vi "Time series ini AVI & header file.vi"(8 "error in (no error)":errorcluster) -> (0 "error out":errorcluster)   [LabVIEW 2017]
uses:
  Typedefs/Channel Selector.ctl
  Global Variables/General Globals.vi
  User Interface/Visualisation/Functional Imaging Viewer/SubVIs/Experiment header interface/Typedefs/Header file type enum.ctl
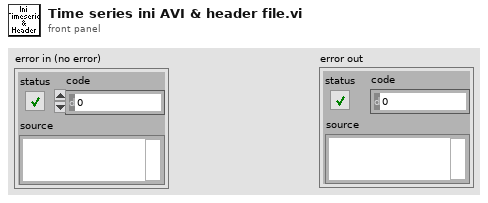
[diagram p1: front panel]
types:
  T1 = typedef "Channel Selector.ctl" = enum16{"Red Channel", "Green Channel", "Blended"}
  T2 = typedef "AOL_Globals.ctl" = cluster{"Imaging Protocol":T3, "Number of POI":u16, "Number of Miniscans":u16, "Number of Trials":u16, "Number of Cycles ":u64, "# Averaged Frames":u16, "Laser power (%)":u8, "Pockels (V)":dbl, "Acquisition Length (sec)":dbl, "Fill time (us)":dbl, "POI Dwell time (us)":dbl, "Miniscan Dwell time per pixel (us)":dbl, "PMT 1":dbl, "PMT 2":dbl, "Back Apperture (mA)":dbl, "Frame Size":T4, "Center Frequency":dbl, "Field of View (norm)":dbl, "DwellTime (us)":dbl, "Wavelength (nm)":dbl, "Zoom":dbl, "AOL Z":dbl, "AOL Mode":T5, "GridXY":dbl, "GridZ":dbl, "TriggerPeriod (sec)":dbl, "Number of Pixels in Miniscan":u16, "Experiment folder path":path, "X centre":dbl, "Y centre":dbl, "Angle (degrees)":dbl, "Plane Mode":T6, "Threshold":u16[], "Regenerate Chirps":bool, "Rectangle ROI length (pixels)":u16, "Rectangle ROI height (pixels)":u16, "AOD fill":u16, "StartupDelay":i32, "Samples Wait after Trigger":u16, "Slip Cycle":u32, "Add Cycle":bool, "Functional Mode":T7, "Z Start":dbl, "Z Stop":dbl, "# Planes":i32}
  T3 = typedef "Imaging Protocols enum.ctl" = enum16{"AOL Z-Stack", "Motor Z Stack", "Functional Acquisition", "Single Plane Acquisition", "Volume Acquisition", "Live Imaging", "Live Plane Imaging", "Live Volume Imaging"}
  T4 = typedef "Frame Size.ctl" = u16
  T5 = typedef "AOL modes.ctl" = enum16{"Raster", "Structural", "Pointing", "Mini Scan", "Alignment"}
  T6 = typedef "Plane Mode.ctl" = u16
  T7 = typedef "Functional Mode.ctl" = enum16{"Point", "Line", "Patch", "Plane", "Volume"}
  T8 = typedef "Header file type enum.ctl" = enum16{"All parameters", "Params for funct acq w ROI or mscn", "Params for funct acq w rectangles", "Live imaging header parameters", "AOL Parameters"}
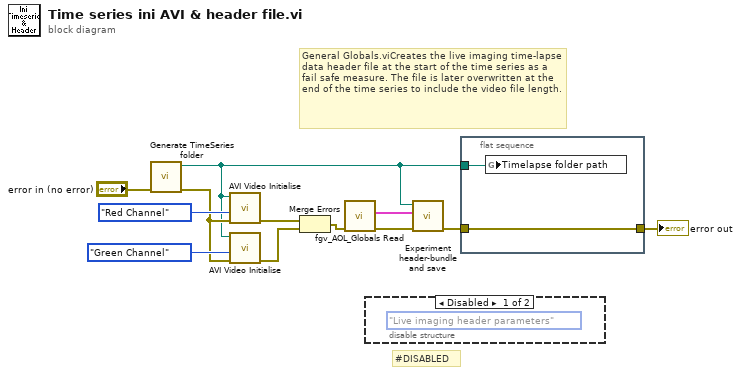
[diagram p0: block diagram]
diagram:
  # "#DISABLED"
  # "General Globals.viCreates the live imaging time-lapse data header file at the start of the time series as a fail safe measure. The file is later overwritten at the end of the time series to include the video file length."
  n1 = call "Generate TimeSeries folder.vi"("error in (no error)"="error in (no error)") -> ("error out"=w3:errorcluster, "Timelapse folder path"=w2:path)  [unwired: 9 in]
  n2 = call "AVI Video Initialise.vi"("error in (no error)"=w3, "Channel"=Channel_Selector."Red Channel", "Timelapse folder path"=w2) -> ("error out"=w11:errorcluster)  [unwired: 8 in]
  n3 = call "AVI Video Initialise.vi"("error in (no error)"=w3, "Channel"=Channel_Selector."Green Channel", "Timelapse folder path"=w2) -> ("error out"=w12:errorcluster)  [unwired: 8 in]
  n4 = Merge Errors(w11, w12) -> (w5:errorcluster)
  n5 = call "fgv_AOL_Globals Read.vi"("error in (no error)"=w5) -> ("error out"=w4:errorcluster, "AOL_Globals"=w1:T2)  [unwired: 8 in, 1 out]
  n6 = disable-structure shown="Disabled" {
    frame Disabled {
      (unwired) Header_file_type_enum."Live imaging header parameters" ("Header file type")
    }
    frame Enabled {
    }
  }
  n7 = call "Experiment header-bundle and save.vi"("error in (no error)"=w4, "AOL_Globals"=w1, "Experiment data folder path"=w2) -> ("error out"=w7:errorcluster)  [unwired: 8 in]
  n8 = flat-sequence {
    tunnel: w7 -> [w14]
    tunnel: [w14] -> w6
    tunnel: w2 -> [w13]
    frame #0 {
      n9 = global write "General Globals.vi" "Timelapse folder path"(w13) -> ()
    }
  }
  "error out" <- w6
